vi "ma_sml_Interpolation by Zero Insert.vi"   [LabVIEW 2020, in "NI_MAPro.lvlib"]
uses:
  NI_MAPro.lvlib
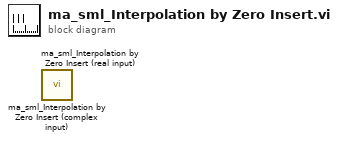
[diagram p0: block diagram]
diagram:
  n1 = call "ma_sml_Interpolation by Zero Insert (complex input).vi"() -> ()  [unwired: 2 in, 1 out]
  n2 = call "ma_sml_Interpolation by Zero Insert (real input).vi"() -> ()  [unwired: 2 in, 1 out]
